vi "Init.vi"(8 "error in (no error)":errorcluster, 11 "Debug":bool) -> (0 "error out":errorcluster, 3 "FileNotFoundException out":refnum<class "FileNotFoundException.lvclass">)   [LabVIEW 2020, in "HTTP Server.lvlib" / "FileNotFoundException.lvclass"]
uses:
  FileNotFoundException.lvclass
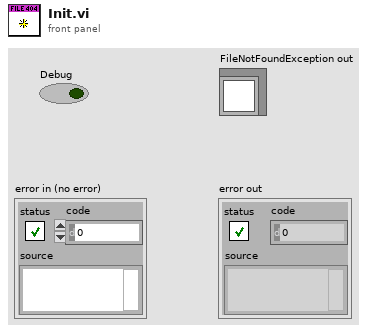
[diagram p1: front panel]
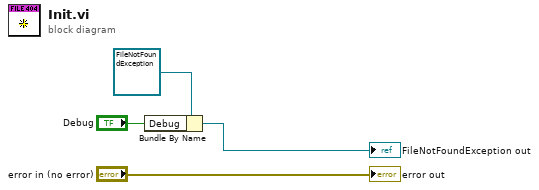
[diagram p0: block diagram]
diagram:
  n1 = Bundle By Name(cluster=refnum<class "FileNotFoundException.lvclass"> refnum ("FileNotFoundException in"), "Debug"="Debug") -> (→"FileNotFoundException out":refnum<class "FileNotFoundException.lvclass">)
  "error out" <- "error in (no error)"
